vi "Get Hardware Data.vi"(11 "Include CPU Info?":bool) -> (3 "Fingerprint":string)   [LabVIEW 2013]
doc: "Generate a hardware fingerprint that is unique for a given system. The fingerprnt includes information about the BIOS and the Mother Board and can include info about the CPU. The function takes considerably longer to retrieve CPU information so this should be taken into account if the user wishes to use this option. The default is to not use the CPU info."
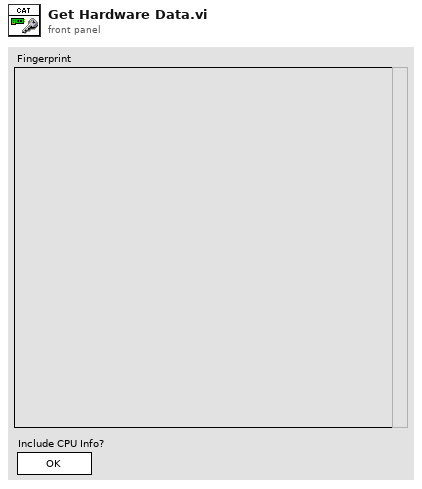
[diagram p1: front panel]
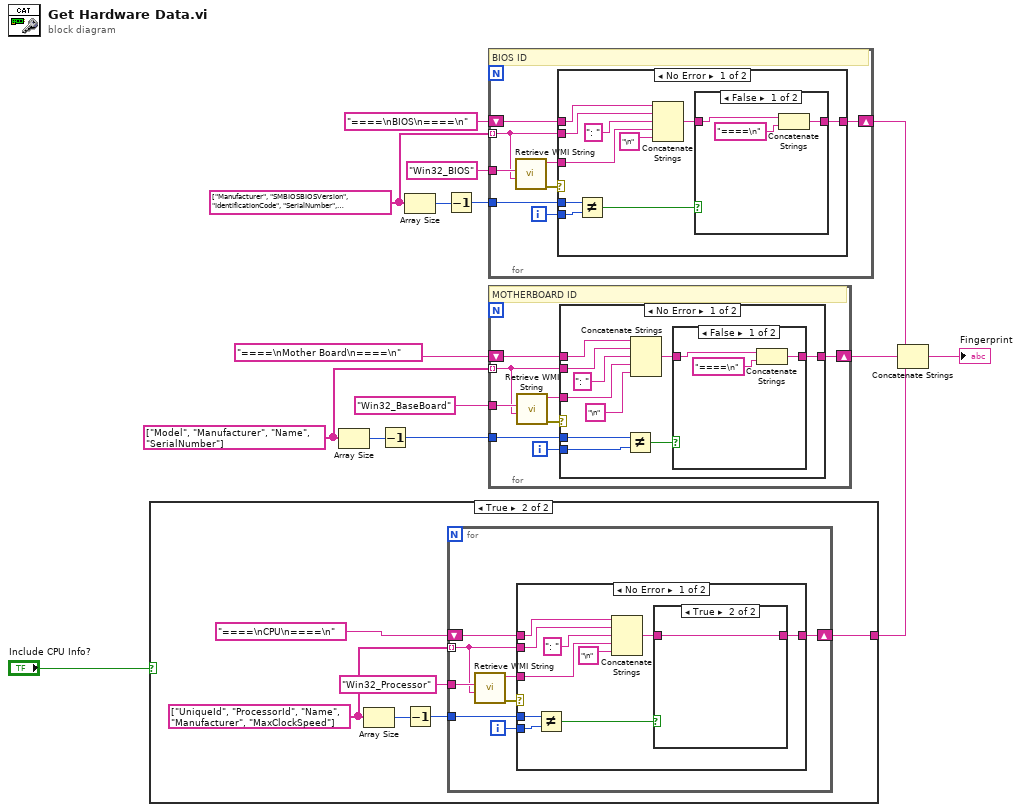
[diagram p0: block diagram]
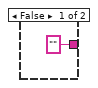
[diagram p2: hidden frame]
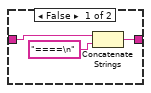
[diagram p3: hidden frame]
diagram:
  w10 = string[] ["Model", "Manufacturer", "Name", "SerialNumber"]
  w5 = string[] ["Manufacturer", "SMBIOSBIOSVersion", "IdentificationCode", "SerialNumber", "ReleaseDate", "Version"]
  n1 = case shown="True" "Include CPU Info?" {
    tunnel: ["" w17] -> w1
    frame False {
    }
    frame True {
      w20 = string[] ["UniqueId", "ProcessorId", "Name", "Manufacturer", "MaxClockSpeed"]
      n2 = Array Size(array=w20) -> (size(s)=w19:i32)
      n3 = Decrement(x=w19) -> (x-1=w18:i32)
      n4 = for {
        tunnel: w20 -> [w23] mode=indexing
        tunnel: "Win32_Processor" ("wmiClass") -> [w30]
        shift-right: [w26] -> w17
        shift-left: "====\nCPU\n====\n" -> [w28]
        tunnel: w18 -> [w24]
        i -> [w25]
        n5 = call "Retrieve WMI String.vi"("wmiProperty"=w23, "wmiClass"=w30) -> ("Error Out"=w29:errorcluster, "LastValue"=w27:string)  [unwired: 7 in, 1 out]
        n6 = case shown="No Error" w29 {
          tunnel: w28 -> [w40 w45]
          tunnel: w27 -> [w32 _]
          tunnel: [w35 w45] -> w26
          tunnel: w25 -> [w39 _]
          tunnel: w24 -> [w38 _]
          tunnel: w23 -> [w34 _]
          frame No Error {
            n7 = Not Equal?(x=w38, y=w39) -> (x != y?=w37:bool)
            n8 = Concatenate Strings(w40, w34, ": " ("string"), w32, "\n" ("string")) -> (w36:string)
            n9 = case shown="True" w37 {
              tunnel: w36 -> [w43 w44]
              tunnel: [w41 w44] -> w35
              frame False {
                n10 = Concatenate Strings(w43, "====\n" ("string")) -> (w41:string)
              }
              frame True {
              }
            }
          }
          frame Error {
          }
        }
      }
    }
  }
  n11 = Array Size(array=w10) -> (size(s)=w9:i32)
  n12 = Decrement(x=w9) -> (x-1=w8:i32)
  n13 = Array Size(array=w5) -> (size(s)=w6:i32)
  n14 = Decrement(x=w6) -> (x-1=w7:i32)
  n15 = for {
    tunnel: w5 -> [w46] mode=indexing
    tunnel: "Win32_BIOS" ("wmiClass") -> [w53]
    shift-right: [w49] -> w13
    shift-left: "====\nBIOS\n====\n" -> [w51]
    tunnel: w7 -> [w47]
    i -> [w48]
    # "BIOS ID"
    n16 = call "Retrieve WMI String.vi"("wmiProperty"=w46, "wmiClass"=w53) -> ("Error Out"=w52:errorcluster, "LastValue"=w50:string)  [unwired: 7 in, 1 out]
    n17 = case shown="No Error" w52 {
      tunnel: w51 -> [w63 w68]
      tunnel: w50 -> [w55 _]
      tunnel: [w58 w68] -> w49
      tunnel: w48 -> [w62 _]
      tunnel: w47 -> [w61 _]
      tunnel: w46 -> [w57 _]
      frame No Error {
        n18 = Not Equal?(x=w61, y=w62) -> (x != y?=w60:bool)
        n19 = Concatenate Strings(w63, w57, ": " ("string"), w55, "\n" ("string")) -> (w59:string)
        n20 = case shown="False" w60 {
          tunnel: w59 -> [w66 w67]
          tunnel: [w64 w67] -> w58
          frame False {
            n21 = Concatenate Strings(w66, "====\n" ("string")) -> (w64:string)
          }
          frame True {
          }
        }
      }
      frame Error {
      }
    }
  }
  n22 = for {
    tunnel: w10 -> [w69] mode=indexing
    tunnel: "Win32_BaseBoard" ("wmiClass") -> [w76]
    shift-right: [w72] -> w14
    shift-left: "====\nMother Board\n====\n" -> [w74]
    tunnel: w8 -> [w70]
    i -> [w71]
    # "MOTHERBOARD ID"
    n23 = call "Retrieve WMI String.vi"("wmiProperty"=w69, "wmiClass"=w76) -> ("Error Out"=w75:errorcluster, "LastValue"=w73:string)  [unwired: 7 in, 1 out]
    n24 = case shown="No Error" w75 {
      tunnel: w74 -> [w86 w91]
      tunnel: w73 -> [w78 _]
      tunnel: [w81 w91] -> w72
      tunnel: w71 -> [w85 _]
      tunnel: w70 -> [w84 _]
      tunnel: w69 -> [w80 _]
      frame No Error {
        n25 = Not Equal?(x=w84, y=w85) -> (x != y?=w83:bool)
        n26 = Concatenate Strings(w86, w80, ": " ("string"), w78, "\n" ("string")) -> (w82:string)
        n27 = case shown="False" w83 {
          tunnel: w82 -> [w89 w90]
          tunnel: [w87 w90] -> w81
          frame False {
            n28 = Concatenate Strings(w89, "====\n" ("string")) -> (w87:string)
          }
          frame True {
          }
        }
      }
      frame Error {
      }
    }
  }
  n29 = Concatenate Strings(w13, w14, w1) -> (→"Fingerprint":string)
